vi "NET_Drive_Motion Profile.vi"(8 "Error":errorcluster, 9 "Read(F) Write(T)":bool=TRUE, 11 "Motion Profile":T1) -> (0 "Error Out":errorcluster, 3 "Motion Profile Out":T1)   [LabVIEW 2017]
uses:
  RoboRio code/TypeDef/CLUSTER_Drive_Motion Profile Arrays.ctl
  RoboRio code/TypeDef/CLUSTER_Drive_Point Specification.ctl
  <vilib>/Rock Robotics/Network Tables/NT Read String Array.vi
  <vilib>/Rock Robotics/Network Tables/NT Write String Array.vi
  <vilib>/Utility/Data Type/NI_Data Type.lvlib
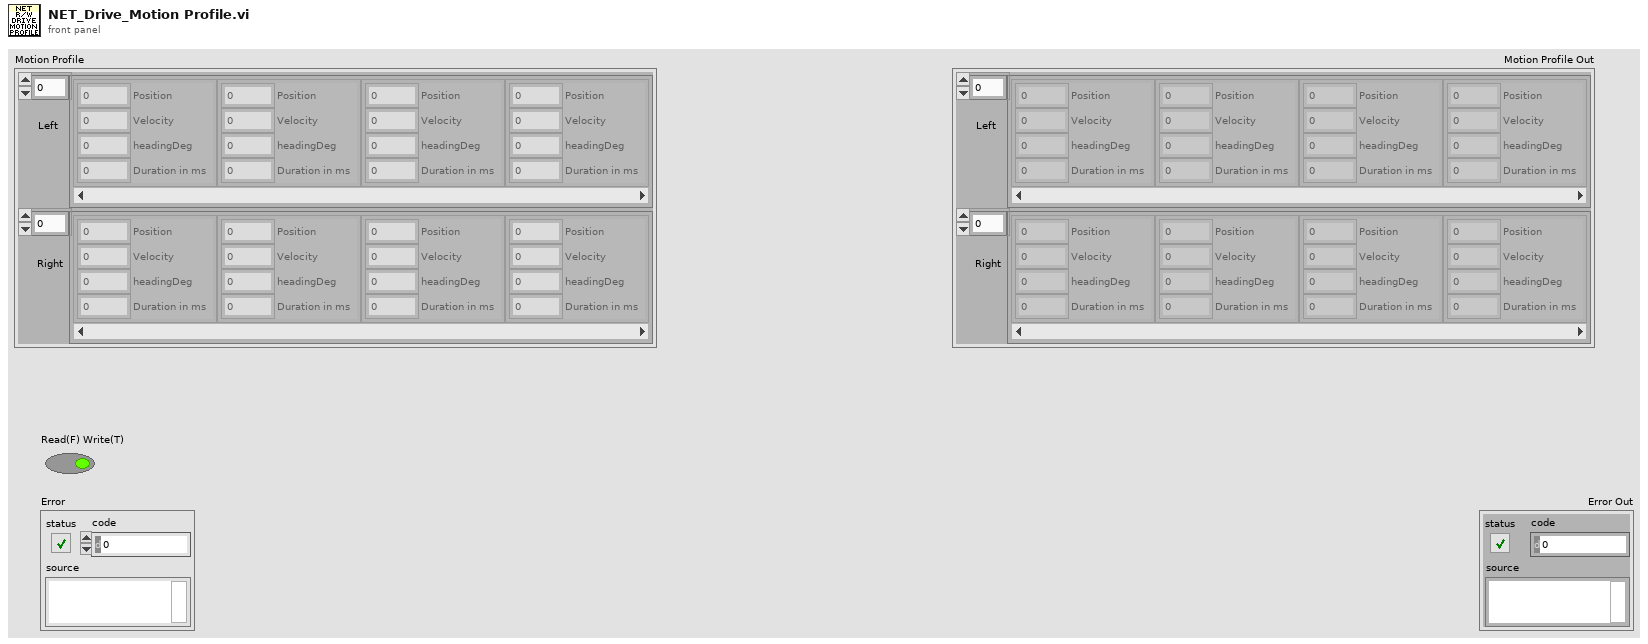
[diagram p1: front panel]
types:
  T1 = typedef "CLUSTER_Drive_Motion Profile Arrays.ctl" = cluster{"Left":T2[], "Right":T2[]}
  T2 = typedef "CLUSTER_Drive_Point Specification.ctl" = cluster{"Position":dbl, "Velocity":dbl, "headingDeg":dbl, "Duration in ms":i32}
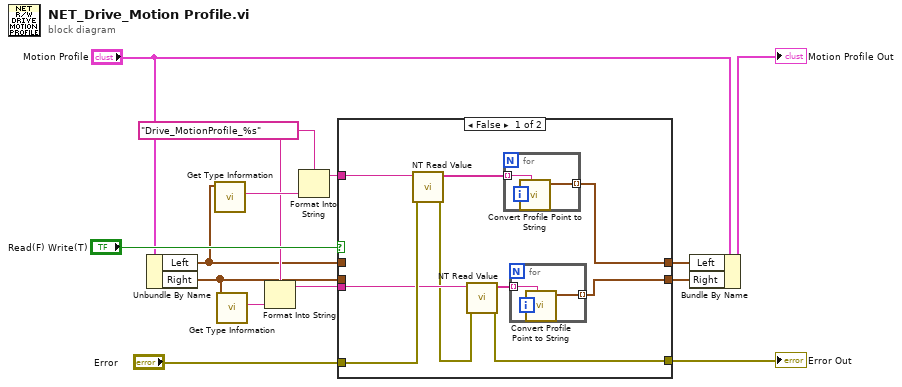
[diagram p0: block diagram]
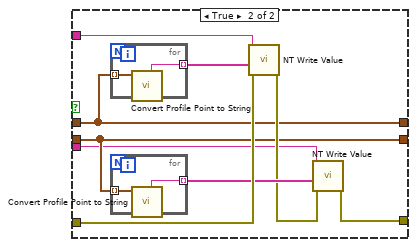
[diagram p2: hidden frame]
diagram:
  w9 = "Drive_MotionProfile_%s" ("Name")
  n1 = Unbundle By Name("Motion Profile") -> ("Left"=w6:T2[], "Right"=w5:T2[])
  n2 = call <vilib>:"Get Type Information.vi"("Variant"=w6) -> ("Name"=w11:string)  [unwired: 6 in, 4 out]
  n3 = call <vilib>:"Get Type Information.vi"("Variant"=w5) -> ("Name"=w8:string)  [unwired: 6 in, 4 out]
  n4 = Format Into String(format string=w9, w8) -> (resulting string=w7:string)  [unwired: 2 in, 1 out]
  n5 = Format Into String(format string=w9, w11) -> (resulting string=w10:string)  [unwired: 2 in, 1 out]
  n6 = case shown="False" "Read(F) Write(T)" {
    tunnel: w10 -> [w23 w36]
    tunnel: [w15 w31] -> w13
    tunnel: "Error" -> [w21 w34]
    tunnel: w7 -> [w17 w28]
    tunnel: w6 -> [_ w30]
    tunnel: w5 -> [_ w29]
    tunnel: [w20 w30] -> w2
    tunnel: [w18 w29] -> w1
    frame False {
      n7 = call-poly <vilib>:"NT Read Value.vi"("error in"=w21, "Name"=w23) -> ("error out"=w16:errorcluster, "String Array"=w22:string[])  [unwired: 8 in]
      n8 = call-poly <vilib>:"NT Read Value.vi"("error in"=w16, "Name"=w17) -> ("error out"=w15:errorcluster, "String Array"=w19:string[])  [unwired: 8 in]
      n9 = for {
        tunnel: w22 -> [w27] mode=indexing
        tunnel: [w26] -> w20 mode=indexing
        n10 = call "Convert Profile Point to String.vi"("Point String"=w27) -> ("Point Cluster Out"=w26:T2)  [unwired: 9 in, 1 out]
      }
      n11 = for {
        tunnel: w19 -> [w25] mode=indexing
        tunnel: [w24] -> w18 mode=indexing
        n12 = call "Convert Profile Point to String.vi"("Point String"=w25) -> ("Point Cluster Out"=w24:T2)  [unwired: 9 in, 1 out]
      }
    }
    frame True {
      n13 = for {
        tunnel: w30 -> [w40] mode=indexing
        tunnel: [w39] -> w35 mode=indexing
        n14 = call "Convert Profile Point to String.vi"("Point Cluster"=w40) -> ("Point String Out"=w39:string)  [unwired: 9 in, 1 out]
      }
      n15 = for {
        tunnel: w29 -> [w38] mode=indexing
        tunnel: [w37] -> w33 mode=indexing
        n16 = call "Convert Profile Point to String.vi"("Point Cluster"=w38) -> ("Point String Out"=w37:string)  [unwired: 9 in, 1 out]
      }
      n17 = call-poly <vilib>:"NT Write Value.vi"("error in"=w34, "String Array"=w35, "Name"=w36) -> ("error out"=w32:errorcluster)  [unwired: 8 in]
      n18 = call-poly <vilib>:"NT Write Value.vi"("error in"=w32, "String Array"=w33, "Name"=w28) -> ("error out"=w31:errorcluster)  [unwired: 8 in]
    }
  }
  "Error Out" <- w13
  n19 = Bundle By Name(cluster="Motion Profile", "Left"=w2, "Right"=w1) -> (→"Motion Profile Out":T1)
